vi "Target Logging.vi"(6 "rt fifo":refnum<k33>) -> (0 "Stop Loop":bool)   [LabVIEW 2018]
uses:
  Target Sensors.ctl
  Target Logging Cluster.ctl
  Target Controller Signals Cluster.ctl
  Logging Data Cluster.ctl
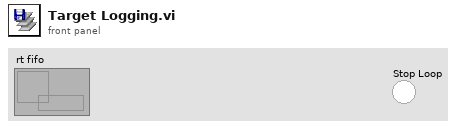
[diagram p1: front panel]
types:
  T1 = typedef "Target Logging Cluster.ctl" = cluster{"Valid for Logging?":bool, "Data":T2}
  T2 = typedef "Logging Data Cluster.ctl" = cluster{"Target Sensors":T3, "Controller Signals":T4}
  T3 = typedef "Target Sensors.ctl" = cluster{"Raw Cable Force (N)":dbl, "Prosthesis Angle (deg)":dbl, "Motor Current (A)":dbl, "Motor Velocity (deg/s)":dbl, "Motor Position (deg)":dbl, "Main Clock Line (s)":dbl, "Filtered Cable Force (N)":dbl}
  T4 = typedef "Target Controller Signals Cluster.ctl" = cluster{"Joint Torque Setpoint (Nm)":dbl, "Cable Force Setpoint (N)":dbl, "Motor Command (deg/s)":dbl, "Filtered Ankle Angle (deg)":dbl}
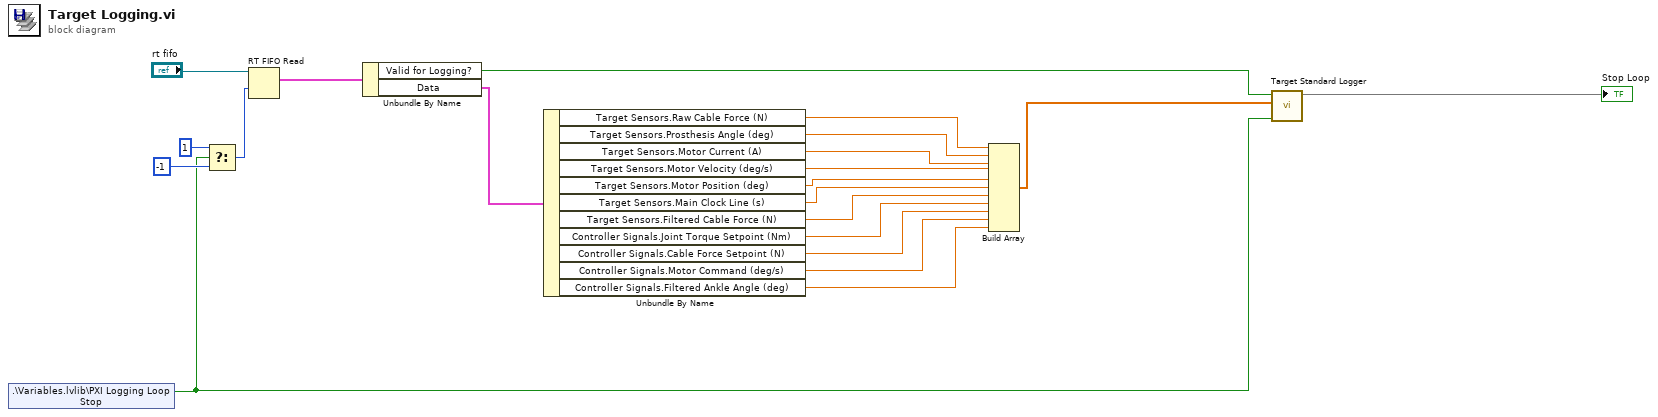
[diagram p0: block diagram]
diagram:
  n1 = shared-variable ".\\Variables.lvlib\\PXI Logging Loop Stop"() -> (w14:bool)  [unwired: 1 in, 1 out]
  n2 = Select(t=1, s=w14, f=-1) -> (s? t:f=w19:i32)
  n3 = RT FIFO Read(0:"rt fifo", 2:w19) -> (9:w16:T1)  [unwired: 2 in, 4 out]
  n4 = Unbundle By Name(w16) -> ("Valid for Logging?"=w15:bool, "Data"=w13:T2)
  n5 = Unbundle By Name(w13) -> ("Target Sensors.Raw Cable Force (N)"=w12:dbl, "Target Sensors.Prosthesis Angle (deg)"=w11:dbl, "Target Sensors.Motor Current (A)"=w10:dbl, "Target Sensors.Motor Velocity (deg/s)"=w9:dbl, "Target Sensors.Motor Position (deg)"=w8:dbl, "Target Sensors.Main Clock Line (s)"=w7:dbl, "Target Sensors.Filtered Cable Force (N)"=w6:dbl, "Controller Signals.Joint Torque Setpoint (Nm)"=w5:dbl, "Controller Signals.Cable Force Setpoint (N)"=w4:dbl, "Controller Signals.Motor Command (deg/s)"=w3:dbl, "Controller Signals.Filtered Ankle Angle (deg)"=w2:dbl)
  n6 = Build Array(w12, w11, w10, w9, w8, w7, w6, w5, w4, w3, w2) -> (w1:dbl[])
  n7 = call "Target Standard Logger.vi"("Stop Command"=w14, "Incoming Data Array"=w1, "Valid for Logging?"=w15) -> (3:→"Stop Loop")  [unwired: 7 in, 1 out]
